vi "TwoCameraDisplayPanel.vi"() -> ()   [LabVIEW 2013]
uses:
  MvLVLib/MvCameraControl.lvlib
  MvLVLib/VIs/CreateGigEHandle.vi
  MvLVLib/VIs/CreateU3VHandle.vi
  <vilib>/picture/picture.llb/imagedata.ctl
panel:
  out "GenTLDeviceArray":T1(array[cluster])
  in  "image data 2":T2 caption="图像数据"
  in  "Rectangle 2":T3
  out "pFrameInfoEx out 2":T4
  in  "pConvertInfo In 2":T5
  out "nWidth 2":u32
  out "nHeight 2":u32
  out "PayloadSize 2":u32
  out "PixelFormat 2":u32
  out "handle out 2":u64
  in  "handle 2":u64
  out "Picture 2":picture
  in  "Device List 2":u16(ring)
  out "U3VDeviceArray":T6(array[cluster])
  out "GigEDeviceArray":T7(array[cluster])
  in  "pConvertInfo In":T5
  out "PixelFormat":u32
  out "handle out":u64
  in  "handle":u64
  in  "Rectangle":T3
  in  "image data":T2 caption="图像数据"
  out "Picture":picture
  out "PayloadSize":u32
  out "pFrameInfoEx out":T4
  out "nHeight":u32
  out "nWidth":u32
  out "Acquisision Flag":bool
  in  "Trigger Mode":bool
  in  "Continuous":bool
  out "打开标志":bool
  in  "stop":bool
  in  "Trigger Once":bool
  in  "Stop":bool
  in  "Start":bool
  in  "Open Device":bool
  in  "Close Device":bool
  in  "Refresh Devices":bool
  in  "Device List":u16(ring)
  # "Initialize"
  # "Acquisition"
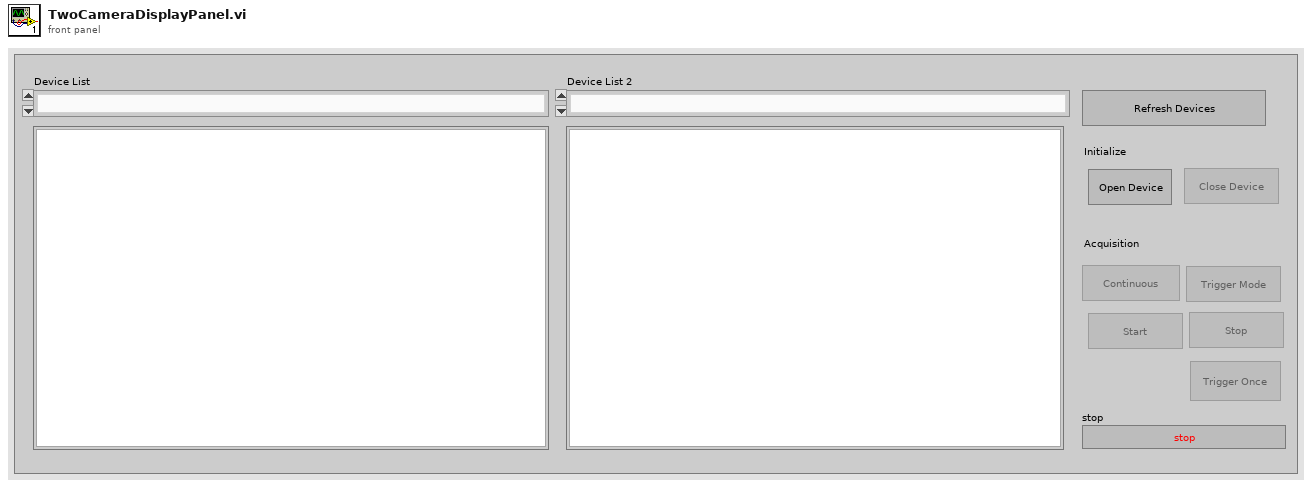
[diagram p1: front panel]
types:
  T1 = cluster{"nMajorVer":u16, "nMinorVer":u16, "nMacAddrHigh":u32, "nMacAddrLow":u32, "nTLayerType":u32, "nReserved0":u32, "nReserved1":u32, "nReserved2":u32, "nReserved3":u32, "chInterfaceID":string, "chVendorName":string, "chModelName":string, "chManufacturerInfo":string, "chDeviceVersion":string, "chSerialNumber":string, "chUserDefinedName":string, "chDeviceID":string, "nRes0":u32, "nRes1":u32, "nRes2":u32, "nRes3":u32, "nRes4":u32, "nRes5":u32, "nRes6":u32}[]
  T2 = typedef "imagedata.ctl" = cluster{"image type":i32, "image depth":i32, "image":u8[], "mask":u8[], "colors":u32[], "Rectangle":cluster{"left":i16, "top":i16, "right":i16, "bottom":i16}}
  T3 = cluster{"left":i16, "top":i16, "right":i16, "bottom":i16}
  T4 = cluster{"nWidth":u16, "nHeight":u16, "enPixelType":i32, "nFrameNum":u32, "nDevTimeStampHigh":u32, "nDevTimeStampLow":u32, "nReserved0":u32, "nHostTimeStamp":i64, "nFrameLen":u32, "nSecondCount]":u32, "nCycleCount":u32, "nCycleOffset":u32, "fGain":u32, "fExposureTime":u32, "nAverageBrightness":u32, "nRed":u32, "nGreen":u32, "nBlue":u32, "nFrameCounter":u32, "nTriggerIndex":u32, "nInput":u32, "nOutput":u32, "nOffsetX":u32, "nOffsetY":u32, "nReserved[0]":u32, "nReserved[1]":u32, "nReserved[2]":u32, "nReserved[3]":u32, "nReserved[4]":u32, "nReserved[5]":u32, "nReserved[6]":u32, "nReserved[7]":u32, "nReserved[8]":u32, "nReserved[9]":u32, "nReserved[10]":u32, "nReserved[11]":u32, "nReserved[12]":u32, "nReserved[13]":u32, "nReserved[14] 10":u32, "nReserved[15] 11":u32, "nReserved[16] 12":u32, "nReserved[17] 13":u32, "nReserved[18] 14":u32, "nReserved[19] 15":u32, "nReserved[20] 16":u32, "nReserved[21] 17":u32, "nReserved[22] 18":u32, "nReserved[23] 19":u32, "nReserved[24] 20":u32, "nReserved[25] 21":u32, "nReserved[26] 22":u32, "nReserved[27] 23":u32, "nReserved[28] 24":u32, "nReserved[29] 25":u32, "nReserved[30] 26":u32, "nReserved[31] 27":u32, "nReserved[32] 28":u32, "nReserved[33] 29":u32, "nReserved[34] 30":u32, "nReserved[35] 31":u32, "nReserved[36] 32":u32, "nReserved[37] 33":u32, "nReserved[38] 34":u32, "nReserved[39] 35":u32, "nReserved[40] 36":u32}
  T5 = cluster{"nWidth":u16, "nHeight":u16, "enSrcPixelType":u32, "nSrcDataLen":u32, "enDstPixelType":u32, "nDstLen":u32, "nDstBufferSize":u32, "nRes0":u32, "nRes1":u32, "nRes2":u32, "nRes3":u32}
  T6 = cluster{"nMajorVer":u16, "nMinorVer":u16, "nMacAddrHigh":u32, "nMacAddrLow":u32, "nTLayerType":u32, "nReserved0":u32, "nReserved1":u32, "nReserved2":u32, "nReserved3":u32, "CrtlInEndPoint":u8, "CrtlOutEndPoint":u8, "StreamEndPoint":u8, "EventEndPoint":u8, "idVendor":u16, "idProduct":u16, "nDeviceNumber":u32, "chDeviceGUID":string, "chVendorName":string, "chModelName":string, "chFamilyName":string, "chDeviceVersion":string, "chManufacturerName":string, "chSerialNumber":string, "chUserDefinedName":string, "nbcdUSB":u32, "nDeviceAddress":u32, "nRes0":u32, "nRes1":u32, "nResAlign":u32}[]
  T7 = cluster{"nMajorVer":u16, "nMinorVer":u16, "nMacAddrHigh":u32, "nMacAddrLow":u32, "nTLayerType":u32, "nReserved0":u32, "nReserved1":u32, "nReserved2":u32, "nReserved3":u32, "nIpCfgOption":u32, "nIpCfgCurrent":u32, "nCurrentIp":u32, "nCurrentSubNetMask":u32, "nDefaultGateWay":u32, "chManualfacturerName":string, "chModelName":string, "chDeviceVersion":string, "chManufacturerSpecificInfo":string, "chSerialNumber":string, "chUserDefinedName":string, "nNetExport":u32, "nRes0":u32, "nRes1":u32, "nRes2":u32, "nRes3":u32}[]
  T8 = enum8{"Enabled", "Disabled", "Disabled and Grayed Out"}
  T9 = cluster{"nMajorVer":u16, "nMinorVer":u16, "nMacAddrHigh":u32, "nMacAddrLow":u32, "nTLayerType":u32, "nReserved0":u32, "nReserved1":u32, "nReserved2":u32, "nReserved3":u32, "nIpCfgOption":u32, "nIpCfgCurrent":u32, "nCurrentIp":u32, "nCurrentSubNetMask":u32, "nDefaultGateWay":u32, "chManualfacturerName":string, "chModelName":string, "chDeviceVersion":string, "chManufacturerSpecificInfo":string, "chSerialNumber":string, "chUserDefinedName":string, "nNetExport":u32, "nRes0":u32, "nRes1":u32, "nRes2":u32, "nRes3":u32}
  T10 = cluster{"nMajorVer":u16, "nMinorVer":u16, "nMacAddrHigh":u32, "nMacAddrLow":u32, "nTLayerType":u32, "nReserved0":u32, "nReserved1":u32, "nReserved2":u32, "nReserved3":u32, "CrtlInEndPoint":u8, "CrtlOutEndPoint":u8, "StreamEndPoint":u8, "EventEndPoint":u8, "idVendor":u16, "idProduct":u16, "nDeviceNumber":u32, "chDeviceGUID":string, "chVendorName":string, "chModelName":string, "chFamilyName":string, "chDeviceVersion":string, "chManufacturerName":string, "chSerialNumber":string, "chUserDefinedName":string, "nbcdUSB":u32, "nDeviceAddress":u32, "nRes0":u32, "nRes1":u32, "nResAlign":u32}
  T11 = cluster{"nMajorVer":u16, "nMinorVer":u16, "nMacAddrHigh":u32, "nMacAddrLow":u32, "nTLayerType":u32, "nReserved0":u32, "nReserved1":u32, "nReserved2":u32, "nReserved3":u32, "chInterfaceID":string, "chVendorName":string, "chModelName":string, "chManufacturerInfo":string, "chDeviceVersion":string, "chSerialNumber":string, "chUserDefinedName":string, "chDeviceID":string, "nRes0":u32, "nRes1":u32, "nRes2":u32, "nRes3":u32, "nRes4":u32, "nRes5":u32, "nRes6":u32}
  T12 = cluster{"nCurValue":u32, "nMax":u32, "nMin":u32, "nInc":u32, "nReserved[0]":u32, "nReserved[1]":u32, "nReserved[2]":u32, "nReserved[3]":u32}
  T13 = cluster{"nCurValue":u32, "nSupportedNum":u32, "nSupportValue":u32[], "nReserved[0]":u32, "nReserved[1]":u32, "nReserved[2]":u32, "nReserved[3]":u32}
  T14 = cluster{"nWidth":u32, "nHeight":u32, "enSrcPixelType":u32, "nSrcDataLen":u32, "enDstPixelType":u32, "nDstLen":u32, "nDstBufferSize":u32, "nRes0":u32, "nRes1":u32, "nRes2":u32, "nRes3":u32}
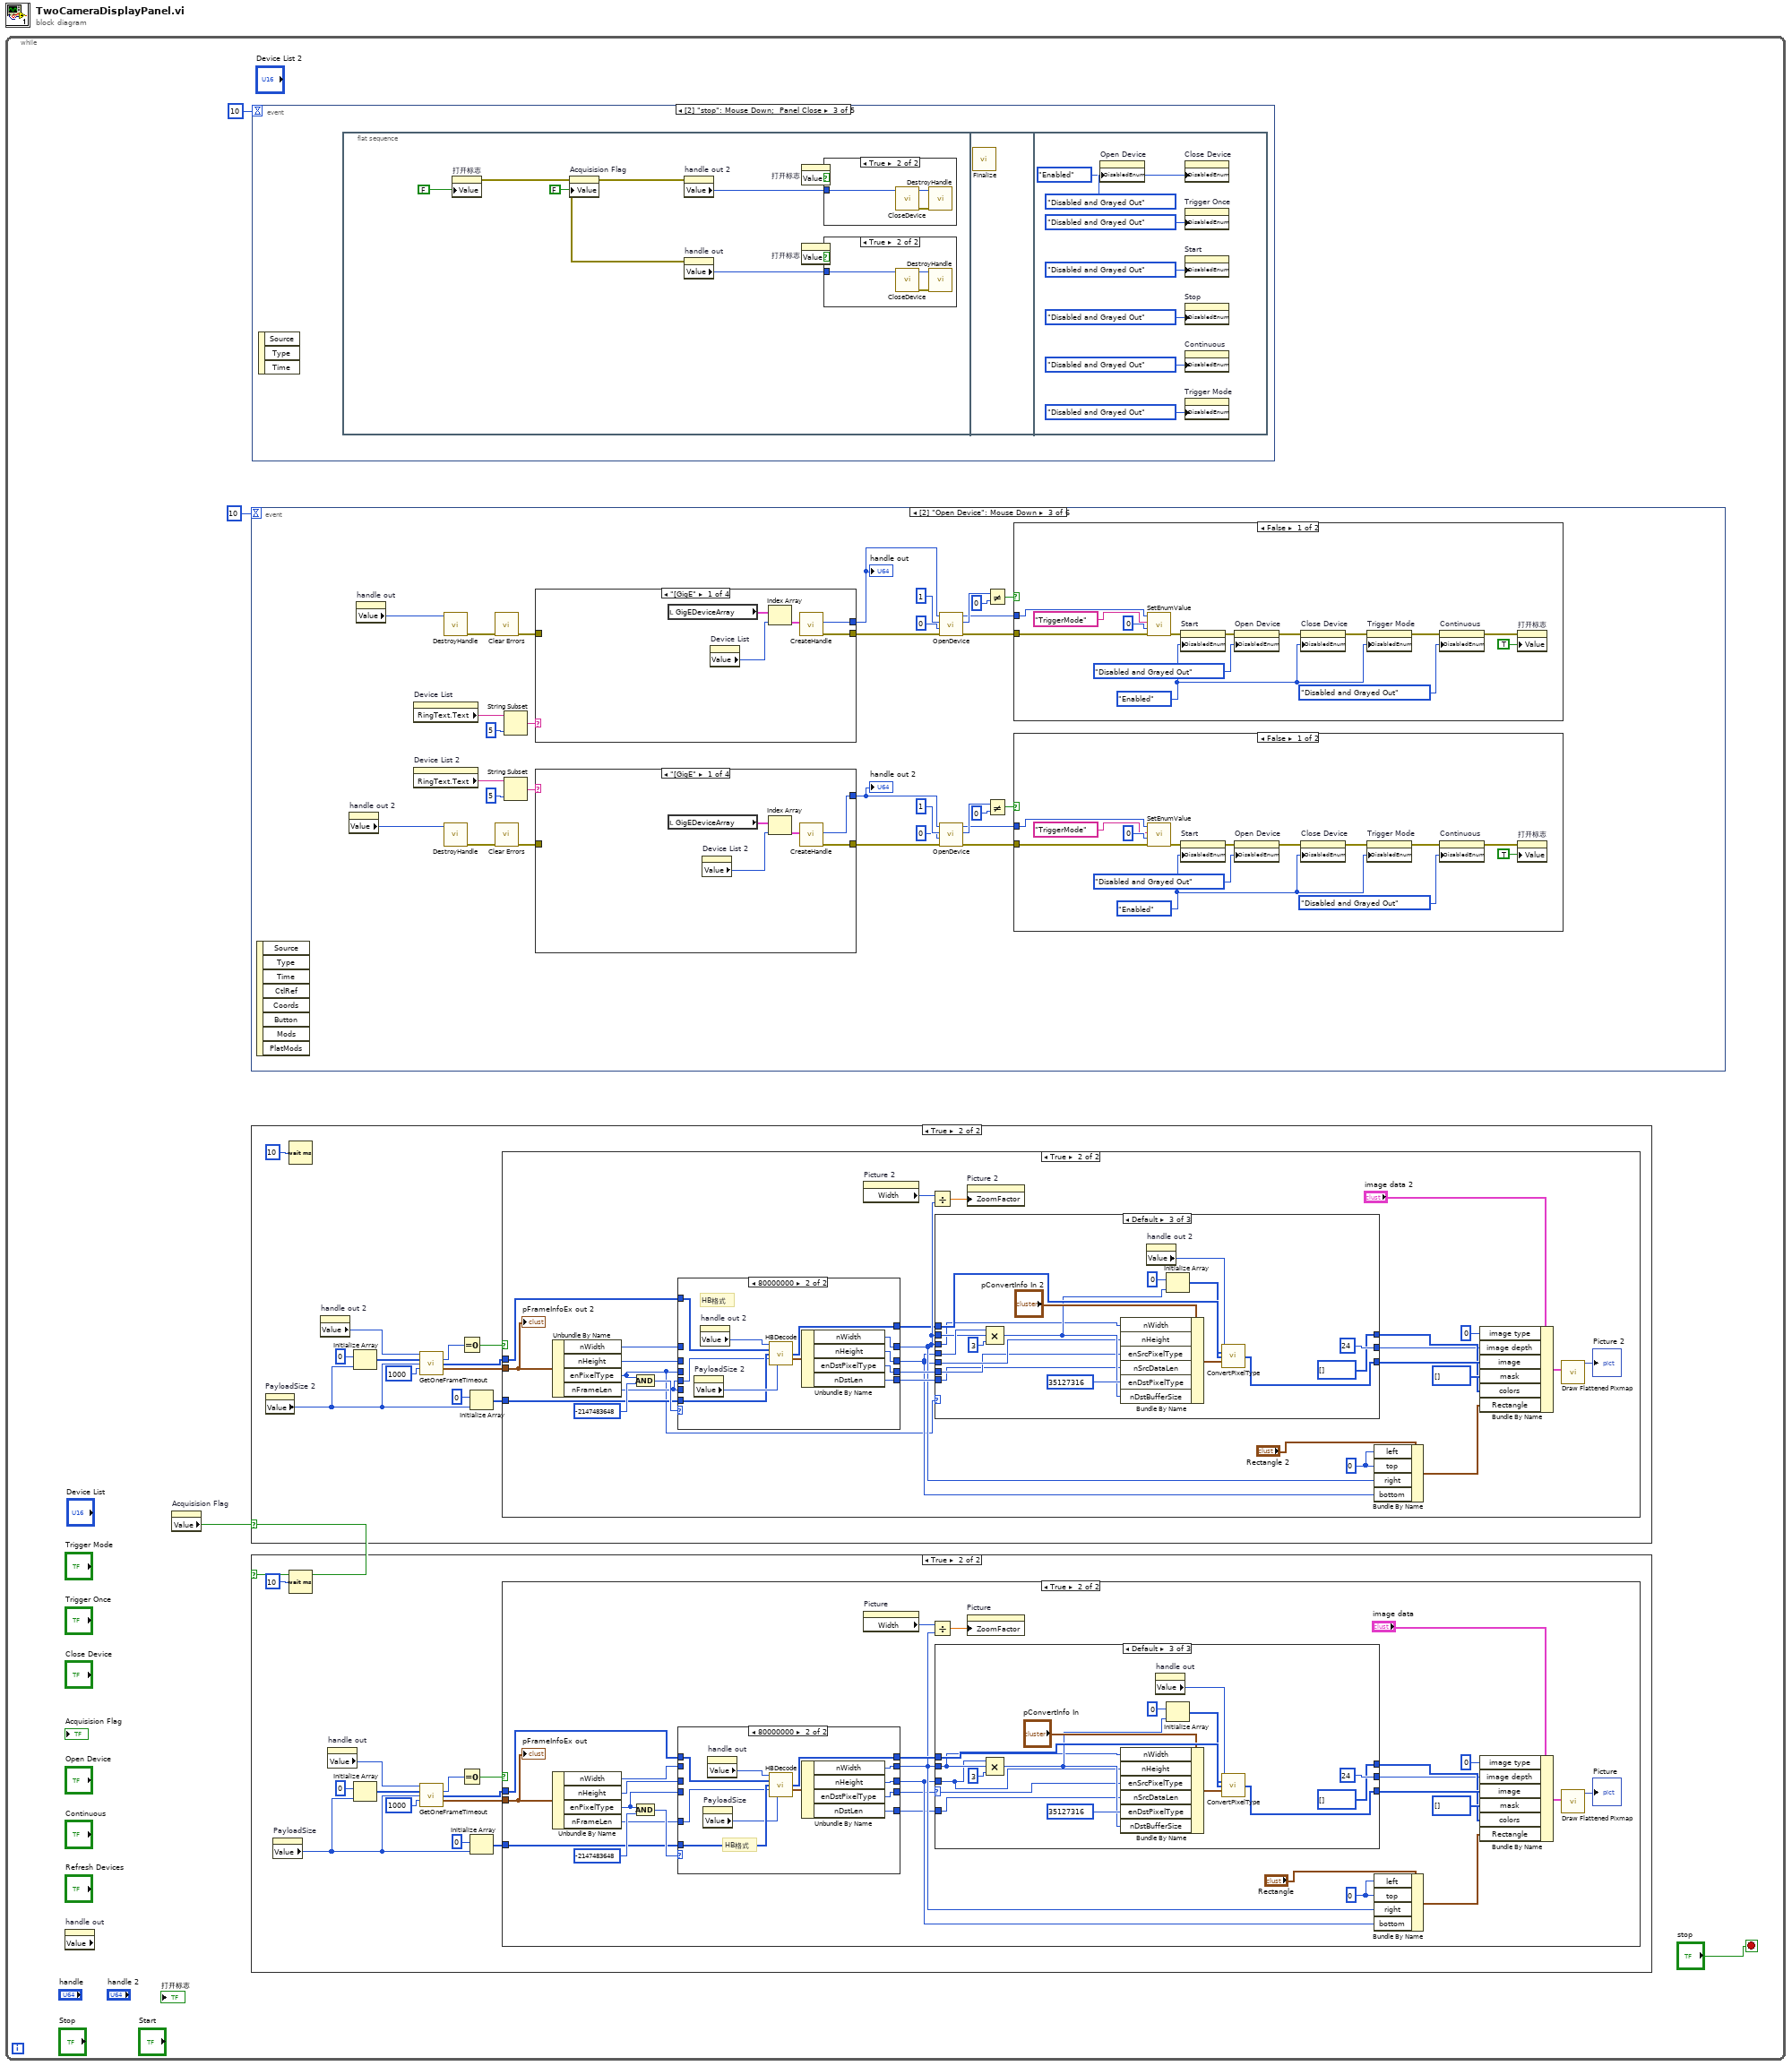
[diagram p0: block diagram]
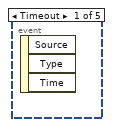
[diagram p2: hidden frame]
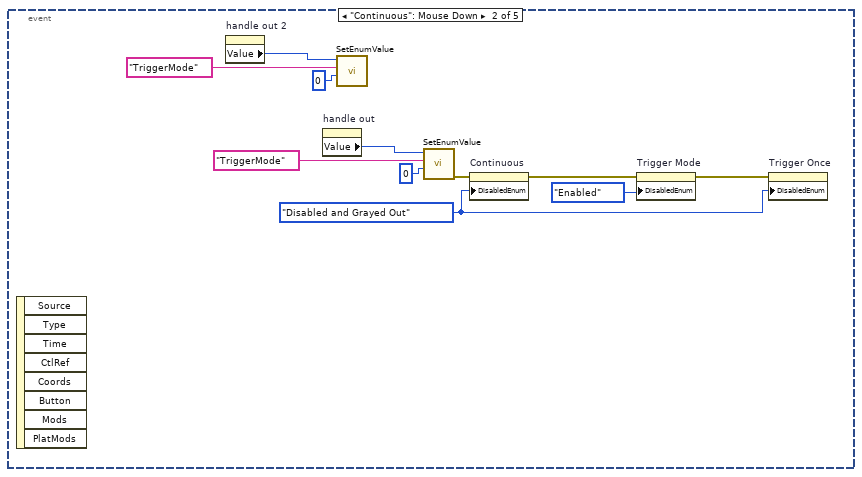
[diagram p3: hidden frame]
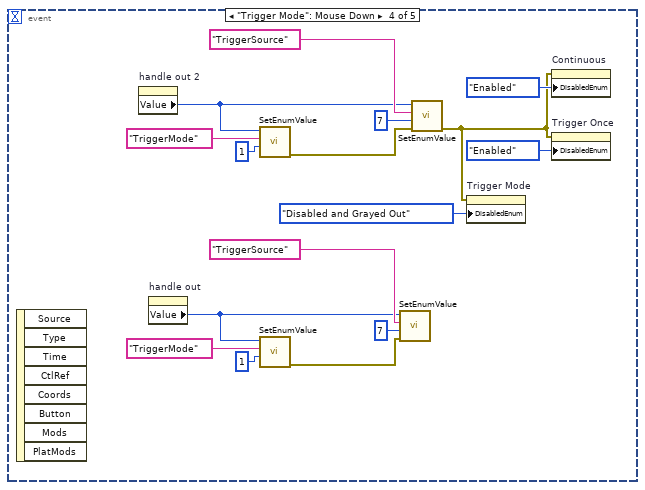
[diagram p6: hidden frame]
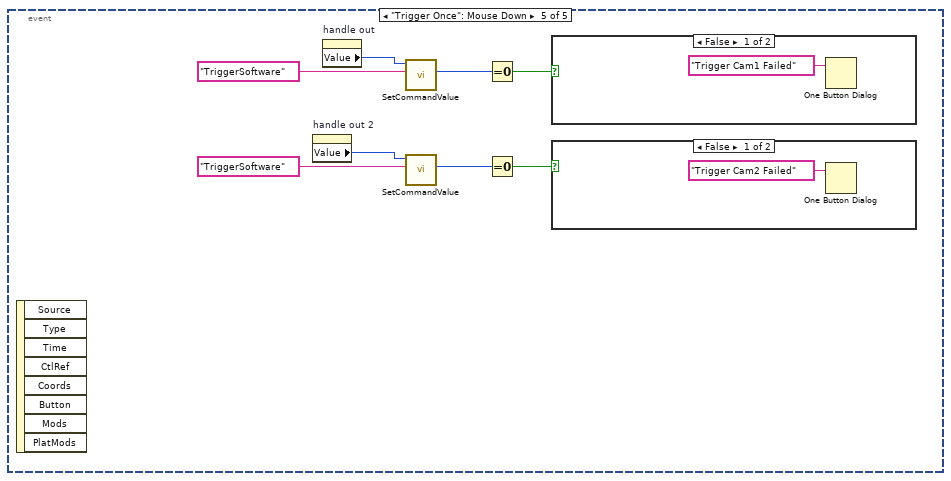
[diagram p7: hidden frame]
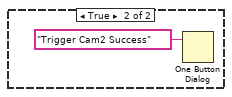
[diagram p8: hidden frame]
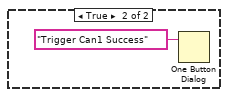
[diagram p9: hidden frame]
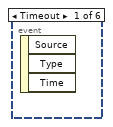
[diagram p10: hidden frame]
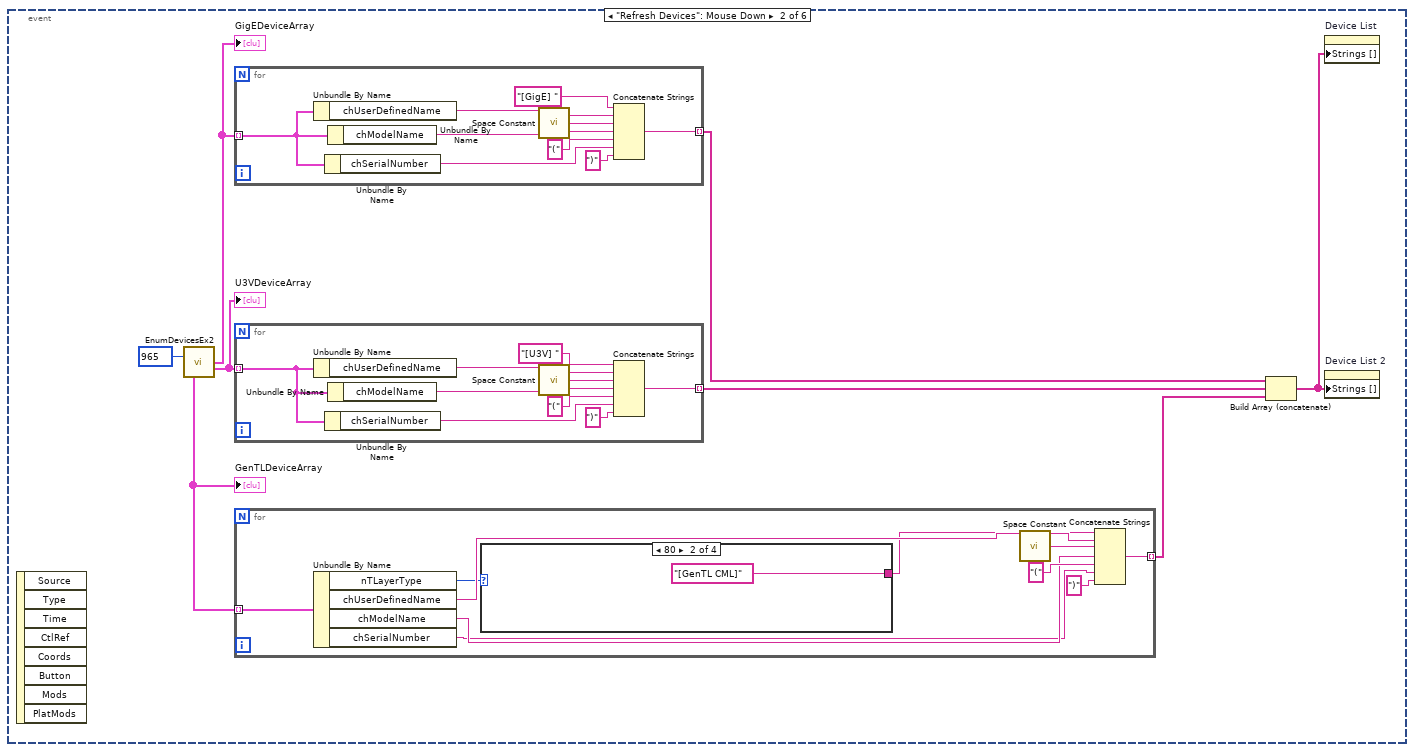
[diagram p11: hidden frame]
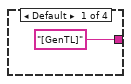
[diagram p12: hidden frame]
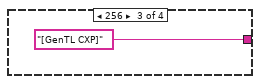
[diagram p13: hidden frame]
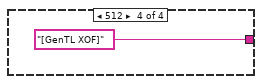
[diagram p14: hidden frame]
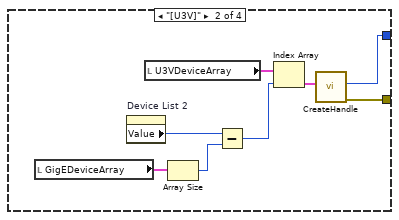
[diagram p15: hidden frame]
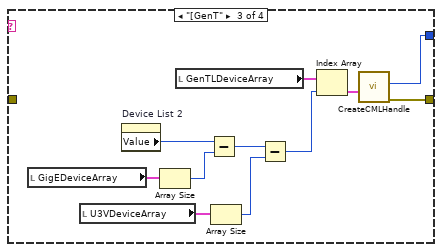
[diagram p16: hidden frame]
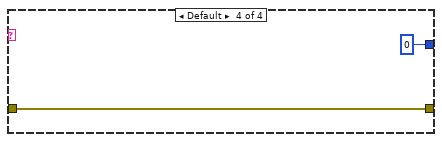
[diagram p17: hidden frame]
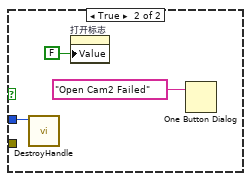
[diagram p18: hidden frame]
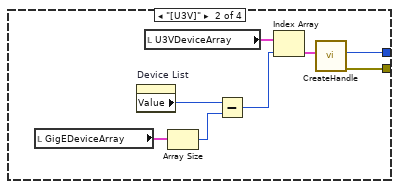
[diagram p19: hidden frame]
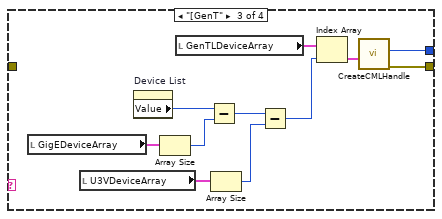
[diagram p20: hidden frame]
diagram:
  n1 = while {
    stop <- "stop" stop-if-true
    n2 = property on="handle out" class="DigNum (strict)" props=["Value"]() -> ()  [unwired: 2 in, 3 out]
    n3 = property on="Acquisision Flag" class="Bool (strict)"() -> ("Value"=w1:bool)  [unwired: 2 in, 2 out]
    n4 = event shown="[2] \"Open Device\": Mouse Down" {
      selector: _ -> [_ _ _ _ _ _]
      dyn-events: _ -> [_ _ _ _ _ _]
      timeout: 10 -> [_ _ _ _ _ _]
      event Timeout {
        n5 = event-data() -> ()  [unwired: 1 in, 3 out]
      }
      event "Refresh Devices": Mouse Down {
        n6 = event-data() -> ()  [unwired: 1 in, 8 out]
        n7 = call "EnumDevicesEx2.vi"("nLayerType"=u32 965) -> ("GigEDeviceArray"=w70:T7, "U3VDeviceArray"=w68:T6, "GenTLDevice"=w67:T1)  [unwired: 9 in, 3 out]
        "GigEDeviceArray" <- w70
        "U3VDeviceArray" <- w68
        "GenTLDeviceArray" <- w67
        n8 = for {
          tunnel: w70 -> [w98] mode=indexing
          tunnel: [w97] -> w65 mode=indexing
          n9 = Unbundle By Name(w98) -> ("chUserDefinedName"=w101:string)
          n10 = Unbundle By Name(w98) -> ("chSerialNumber"=w99:string)
          n11 = Unbundle By Name(w98) -> ("chModelName"=w100:string)
          n12 = call <vilib>:"Space Constant.vi"() -> ("String"=w104:string)
          n13 = Concatenate Strings("[GigE] " ("字符串"), w101, w104, w100, "(" ("字符串"), w99, ")" ("字符串")) -> (w97:string)
        }
        n14 = for {
          tunnel: w68 -> [w91] mode=indexing
          tunnel: [w88] -> w71 mode=indexing
          n15 = Unbundle By Name(w91) -> ("chUserDefinedName"=w95:string)
          n16 = Unbundle By Name(w91) -> ("chSerialNumber"=w90:string)
          n17 = Unbundle By Name(w91) -> ("chModelName"=w93:string)
          n18 = call <vilib>:"Space Constant.vi"() -> ("String"=w94:string)
          n19 = Concatenate Strings("[U3V] " ("字符串"), w95, w94, w93, "(" ("字符串"), w90, ")" ("字符串")) -> (w88:string)
        }
        n20 = for {
          tunnel: w67 -> [w79] mode=indexing
          tunnel: [w77] -> w66 mode=indexing
          n21 = Unbundle By Name(w79) -> ("nTLayerType"=w74:u32, "chUserDefinedName"=w82:string, "chModelName"=w76:string, "chSerialNumber"=w75:string)
          n22 = case shown="80" w74 {
            tunnel: ["[GenTL]" ("字符串") "[GenTL CML]" ("字符串") "[GenTL CXP]" ("字符串") "[GenTL XOF]" ("字符串")] -> w73
            frame Default {
            }
            frame 128 {
            }
            frame 256 {
            }
            frame 512 {
            }
          }
          n23 = call <vilib>:"Space Constant.vi"() -> ("String"=w81:string)
          n24 = Concatenate Strings(w73, w82, w81, w76, "(" ("字符串"), w75, ")" ("字符串")) -> (w77:string)
        }
        n25 = Build Array (concatenate)(w65, w71, w66) -> (w69:string[])
        n26 = property on="Device List" class="Ring (strict)"("Strings []"=w69) -> ()  [unwired: 2 in, 2 out]
        n27 = property on="Device List 2" class="Ring (strict)"("Strings []"=w69) -> ()  [unwired: 2 in, 2 out]
      }
      event "Open Device": Mouse Down {
        n28 = event-data() -> ()  [unwired: 1 in, 8 out]
        n29 = property on="handle out 2" class="DigNum (strict)"() -> ("Value"=w111:u64)  [unwired: 2 in, 2 out]
        n30 = property on="handle out" class="DigNum (strict)"() -> ("Value"=w127:u64)  [unwired: 2 in, 2 out]
        n31 = property on="Device List" class="Ring (strict)"() -> ("RingText.Text"=w124:string)  [unwired: 2 in, 2 out]
        n32 = property on="Device List 2" class="Ring (strict)"() -> ("RingText.Text"=w109:string)  [unwired: 2 in, 2 out]
        n33 = call "DestroyHandle.vi"("handle"=w127) -> ("error out"=w126:errorcluster)  [unwired: 9 in, 1 out]
        n34 = call "DestroyHandle.vi"("handle"=w111) -> ("error out"=w112:errorcluster)  [unwired: 9 in, 1 out]
        n35 = call <vilib>:"Clear Errors.vi"("error in (no error)"=w126) -> ("error out"=w120:errorcluster)  [unwired: 5 in, 1 out]
        n36 = call <vilib>:"Clear Errors.vi"("error in (no error)"=w112) -> ("error out"=w105:errorcluster)  [unwired: 5 in, 1 out]
        n37 = String Subset(string=w124, length (rest)=5 ("长度（剩余）")) -> (substring=w123:string)  [unwired: 1 in]
        n38 = String Subset(string=w109, length (rest)=5 ("长度（剩余）")) -> (substring=w108:string)  [unwired: 1 in]
        n39 = case shown="\"[GigE\"" w123 {
          tunnel: [w181 w187 w199 w203] -> w122
          tunnel: [w180 w186 w198 u64 0 ("handle")] -> w121
          tunnel: w120 -> [_ _ _ w203]
          frame "[GigE" {
            n40 = local read "GigEDeviceArray"() -> (w179:T7)
            n41 = property on="Device List" class="Ring (strict)"() -> ("Value"=w182:u16)  [unwired: 2 in, 2 out]
            n42 = Index Array(array=w179, index=w182) -> (element=w178:T9)
            n43 = call-poly "CreateHandle.vi"("GigEDevice"=w178) -> ("error out"=w181:errorcluster, "handle"=w180:u64)  [unwired: 7 in, 1 out]
          }
          frame "[U3V]" {
            n44 = local read "GigEDeviceArray"() -> (w184:T7)
            n45 = property on="Device List" class="Ring (strict)"() -> ("Value"=w190:u16)  [unwired: 2 in, 2 out]
            n46 = local read "U3VDeviceArray"() -> (w185:T6)
            n47 = Array Size(array=w184) -> (size(s)=w189:i32)
            n48 = Subtract(x=w190, y=w189) -> (x-y=w188:i32)
            n49 = Index Array(array=w185, index=w188) -> (element=w183:T10)
            n50 = call-poly "CreateHandle.vi"("U3VDevice"=w183) -> ("error out"=w187:errorcluster, "handle"=w186:u64)  [unwired: 7 in, 1 out]
          }
          frame "[GenT" {
            n51 = local read "GigEDeviceArray"() -> (w192:T7)
            n52 = local read "U3VDeviceArray"() -> (w191:T6)
            n53 = property on="Device List" class="Ring (strict)"() -> ("Value"=w201:u16)  [unwired: 2 in, 2 out]
            n54 = Array Size(array=w192) -> (size(s)=w200:i32)
            n55 = local read "GenTLDeviceArray"() -> (w197:T1)
            n56 = Subtract(x=w201, y=w200) -> (x-y=w196:i32)
            n57 = Array Size(array=w191) -> (size(s)=w195:i32)
            n58 = Subtract(x=w196, y=w195) -> (x-y=w194:i32)
            n59 = Index Array(array=w197, index=w194) -> (element=w193:T11)
            n60 = call "CreateCMLHandle.vi"("GenTLCMLDevice"=w193) -> ("error out"=w199:errorcluster, "handle"=w198:u64)  [unwired: 7 in, 1 out]
          }
          frame Default {
          }
        }
        "handle out" <- w121
        n61 = case shown="\"[GigE\"" w108 {
          tunnel: [w138 w144 w156 w160] -> w106
          tunnel: [w137 w143 w155 u64 0 ("handle")] -> w107
          tunnel: w105 -> [_ _ _ w160]
          frame "[GigE" {
            n62 = local read "GigEDeviceArray"() -> (w136:T7)
            n63 = property on="Device List 2" class="Ring (strict)"() -> ("Value"=w139:u16)  [unwired: 2 in, 2 out]
            n64 = Index Array(array=w136, index=w139) -> (element=w135:T9)
            n65 = call-poly "CreateHandle.vi"("GigEDevice"=w135) -> ("error out"=w138:errorcluster, "handle"=w137:u64)  [unwired: 7 in, 1 out]
          }
          frame "[U3V]" {
            n66 = local read "GigEDeviceArray"() -> (w141:T7)
            n67 = property on="Device List 2" class="Ring (strict)"() -> ("Value"=w147:u16)  [unwired: 2 in, 2 out]
            n68 = local read "U3VDeviceArray"() -> (w142:T6)
            n69 = Array Size(array=w141) -> (size(s)=w146:i32)
            n70 = Subtract(x=w147, y=w146) -> (x-y=w145:i32)
            n71 = Index Array(array=w142, index=w145) -> (element=w140:T10)
            n72 = call-poly "CreateHandle.vi"("U3VDevice"=w140) -> ("error out"=w144:errorcluster, "handle"=w143:u64)  [unwired: 7 in, 1 out]
          }
          frame "[GenT" {
            n73 = local read "GigEDeviceArray"() -> (w149:T7)
            n74 = local read "U3VDeviceArray"() -> (w148:T6)
            n75 = property on="Device List 2" class="Ring (strict)"() -> ("Value"=w158:u16)  [unwired: 2 in, 2 out]
            n76 = Array Size(array=w149) -> (size(s)=w157:i32)
            n77 = local read "GenTLDeviceArray"() -> (w154:T1)
            n78 = Subtract(x=w158, y=w157) -> (x-y=w153:i32)
            n79 = Array Size(array=w148) -> (size(s)=w152:i32)
            n80 = Subtract(x=w153, y=w152) -> (x-y=w151:i32)
            n81 = Index Array(array=w154, index=w151) -> (element=w150:T11)
            n82 = call "CreateCMLHandle.vi"("GenTLCMLDevice"=w150) -> ("error out"=w156:errorcluster, "handle"=w155:u64)  [unwired: 7 in, 1 out]
          }
          frame Default {
          }
        }
        "handle out 2" <- w107
        n83 = call "OpenDevice.vi"("error in (no error)"=w122, "nSwitchoverKey"=u16 0, "nAccessMode"=u32 1, "handle"=w121) -> ("error out"=w130:errorcluster, "return"=w129:i32, "handle out"=w128:u64)  [unwired: 5 in]
        n84 = call "OpenDevice.vi"("error in (no error)"=w106, "nSwitchoverKey"=u16 0, "nAccessMode"=u32 1, "handle"=w107) -> ("error out"=w115:errorcluster, "return"=w114:i32, "handle out"=w113:u64)  [unwired: 5 in]
        n85 = Not Equal?(x=w129, y=0) -> (x != y?=w133:bool)
        n86 = Not Equal?(x=w114, y=0) -> (x != y?=w118:bool)
        n87 = case shown="False" w133 {
          tunnel: w128 -> [w205 w218]
          tunnel: w130 -> [w206 _]
          frame False {
            w204 = T8."Enabled" ("禁用")
            n88 = call "SetEnumValue.vi"("error in (no error)"=w206, "nValue"=u32 0, "strKey"="TriggerMode", "handle"=w205) -> ("error out"=w216:errorcluster)  [unwired: 5 in, 2 out]
            n89 = property on="Start" class="Bool"(error in=w216, "DisabledEnum"=w204) -> (error out=w214:errorcluster)  [unwired: 1 in, 1 out]
            n90 = property on="Open Device" class="Bool"(error in=w214, "DisabledEnum"=T8."Disabled and Grayed Out" ("禁用")) -> (error out=w213:errorcluster)  [unwired: 1 in, 1 out]
            n91 = property on="Close Device" class="Bool"(error in=w213, "DisabledEnum"=w204) -> (error out=w211:errorcluster)  [unwired: 1 in, 1 out]
            n92 = property on="Trigger Mode" class="Bool"(error in=w211, "DisabledEnum"=w204) -> (error out=w209:errorcluster)  [unwired: 1 in, 1 out]
            n93 = property on="Continuous" class="Bool"(error in=w209, "DisabledEnum"=T8."Disabled and Grayed Out" ("禁用")) -> (error out=w207:errorcluster)  [unwired: 1 in, 1 out]
            n94 = property on="打开标志" class="Bool (strict)"(error in=w207, "Value"=TRUE ("布尔")) -> ()  [unwired: 1 in, 2 out]
          }
          frame True {
            n95 = call "DestroyHandle.vi"("handle"=w218) -> ()  [unwired: 9 in, 2 out]
            n96 = property on="打开标志" class="Bool (strict)"("Value"=FALSE) -> ()  [unwired: 2 in, 2 out]
            n97 = One Button Dialog(message="Open Cam1 Failed") -> ()  [unwired: 1 in, 1 out]
          }
        }
        n98 = case shown="False" w118 {
          tunnel: w113 -> [w162 w175]
          tunnel: w115 -> [w163 _]
          frame False {
            w161 = T8."Enabled" ("禁用")
            n99 = call "SetEnumValue.vi"("error in (no error)"=w163, "nValue"=u32 0, "strKey"="TriggerMode", "handle"=w162) -> ("error out"=w173:errorcluster)  [unwired: 5 in, 2 out]
            n100 = property on="Start" class="Bool"(error in=w173, "DisabledEnum"=w161) -> (error out=w171:errorcluster)  [unwired: 1 in, 1 out]
            n101 = property on="Open Device" class="Bool"(error in=w171, "DisabledEnum"=T8."Disabled and Grayed Out" ("禁用")) -> (error out=w170:errorcluster)  [unwired: 1 in, 1 out]
            n102 = property on="Close Device" class="Bool"(error in=w170, "DisabledEnum"=w161) -> (error out=w168:errorcluster)  [unwired: 1 in, 1 out]
            n103 = property on="Trigger Mode" class="Bool"(error in=w168, "DisabledEnum"=w161) -> (error out=w166:errorcluster)  [unwired: 1 in, 1 out]
            n104 = property on="Continuous" class="Bool"(error in=w166, "DisabledEnum"=T8."Disabled and Grayed Out" ("禁用")) -> (error out=w164:errorcluster)  [unwired: 1 in, 1 out]
            n105 = property on="打开标志" class="Bool (strict)"(error in=w164, "Value"=TRUE ("布尔")) -> ()  [unwired: 1 in, 2 out]
          }
          frame True {
            n106 = call "DestroyHandle.vi"("handle"=w175) -> ()  [unwired: 9 in, 2 out]
            n107 = property on="打开标志" class="Bool (strict)"("Value"=FALSE) -> ()  [unwired: 2 in, 2 out]
            n108 = One Button Dialog(message="Open Cam2 Failed") -> ()  [unwired: 1 in, 1 out]
          }
        }
      }
      event "Close Device": Mouse Down {
        w222 = T8."Disabled and Grayed Out" ("禁用")
        n109 = event-data() -> ()  [unwired: 1 in, 8 out]
        n110 = property on="打开标志" class="Bool (strict)"("Value"=FALSE ("打开标志")) -> (error out=w227:errorcluster)  [unwired: 2 in, 1 out]
        n111 = property on="Acquisision Flag" class="Bool (strict)"(error in=w227, "Value"=FALSE ("采集标志")) -> (error out=w221:errorcluster)  [unwired: 1 in, 1 out]
        n112 = property on="Open Device" class="Bool"("DisabledEnum"=T8."Enabled" ("禁用")) -> (error out=w229:errorcluster)  [unwired: 2 in, 1 out]
        n113 = property on="Close Device" class="Bool"(error in=w229, "DisabledEnum"=w222) -> ()  [unwired: 1 in, 2 out]
        n114 = property on="Start" class="Bool"("DisabledEnum"=w222) -> ()  [unwired: 2 in, 2 out]
        n115 = property on="Stop" class="Bool"("DisabledEnum"=w222) -> ()  [unwired: 2 in, 2 out]
        n116 = property on="Trigger Once" class="Bool"("DisabledEnum"=w222) -> ()  [unwired: 2 in, 2 out]
        n117 = property on="Continuous" class="Bool"("DisabledEnum"=w222) -> ()  [unwired: 2 in, 2 out]
        n118 = property on="Trigger Mode" class="Bool"("DisabledEnum"=w222) -> ()  [unwired: 2 in, 2 out]
        n119 = property on="handle out" class="DigNum (strict)"(error in=w221) -> ("Value"=w223:u64)  [unwired: 1 in, 2 out]
        n120 = property on="handle out 2" class="DigNum (strict)"(error in=w221) -> ("Value"=w231:u64)  [unwired: 1 in, 2 out]
        n121 = call "CloseDevice.vi"("handle"=w223) -> ("error out"=w225:errorcluster, "handle out"=w224:u64)  [unwired: 8 in, 1 out]
        n122 = call "CloseDevice.vi"("handle"=w231) -> ("error out"=w233:errorcluster, "handle out"=w232:u64)  [unwired: 8 in, 1 out]
        n123 = call "DestroyHandle.vi"("error in (no error)"=w225, "handle"=w224) -> ()  [unwired: 8 in, 2 out]
        n124 = call "DestroyHandle.vi"("error in (no error)"=w233, "handle"=w232) -> ()  [unwired: 8 in, 2 out]
      }
      event "Start": Mouse Down {
        n125 = event-data() -> ()  [unwired: 1 in, 8 out]
        n126 = property on="handle out 2" class="DigNum (strict)"() -> ("Value"=w234:u64)  [unwired: 2 in, 2 out]
        n127 = property on="handle out" class="DigNum (strict)"() -> ("Value"=w249:u64)  [unwired: 2 in, 2 out]
        n128 = call "GetIntValue.vi"("strKey"="PayloadSize", "handle"=w234) -> ("error out"=w244:errorcluster, "pIntValue out"=w240:T12, "handle out"=w237:u64)  [unwired: 6 in, 1 out]
        n129 = call "GetIntValue.vi"("strKey"="PayloadSize", "handle"=w249) -> ("error out"=w259:errorcluster, "pIntValue out"=w255:T12, "handle out"=w252:u64)  [unwired: 6 in, 1 out]
        n130 = Unbundle By Name(w240) -> ("nCurValue"=→"PayloadSize 2":u32)
        n131 = Unbundle By Name(w255) -> ("nCurValue"=→"PayloadSize":u32)
        n132 = call "GetEnumValue.vi"("error in (no error)"=w244, "strKey"="PixelFormat", "handle"=w237) -> ("error out"=w243:errorcluster, "pEnumValue out"=w245:T13, "handle out"=w236:u64)  [unwired: 5 in, 1 out]
        n133 = call "GetEnumValue.vi"("error in (no error)"=w259, "strKey"="PixelFormat", "handle"=w252) -> ("error out"=w258:errorcluster, "pEnumValue out"=w260:T13, "handle out"=w251:u64)  [unwired: 5 in, 1 out]
        n134 = Unbundle By Name(w245) -> ("nCurValue"=→"PixelFormat 2":u32)
        n135 = Unbundle By Name(w260) -> ("nCurValue"=→"PixelFormat":u32)
        n136 = call "StartGrabbing.vi"("error in (no error)"=w243, "handle"=w236) -> ("error out"=w242:errorcluster, "function return"=w248:i32, "handle out"=w235:u64)  [unwired: 7 in]
        n137 = call "StartGrabbing.vi"("error in (no error)"=w258, "handle"=w251) -> ("error out"=w257:errorcluster, "function return"=w263:i32, "handle out"=w250:u64)  [unwired: 7 in]
        n138 = Not Equal To 0?(x=w248) -> (x != 0?=w247:bool)
        n139 = Not Equal To 0?(x=w263) -> (x != 0?=w262:bool)
        n140 = case shown="False" w247 {
          tunnel: w234 -> [_ _]
          tunnel: w242 -> [w268 _]
          tunnel: w235 -> [w267 _]
          frame False {
            n141 = call "GetIntValue.vi"("error in (no error)"=w268, "strKey"="Width", "handle"=w267) -> ("error out"=w274:errorcluster, "pIntValue out"=w269:T12, "handle out"=w266:u64)  [unwired: 5 in, 1 out]
            n142 = Unbundle By Name(w269) -> ("nCurValue"=→"nWidth 2":u32)
            n143 = property on="Stop" class="Bool"("DisabledEnum"=T8."Enabled" ("禁用")) -> (error out=w270:errorcluster)  [unwired: 2 in, 1 out]
            n144 = property on="Continuous" class="Bool"(error in=w270) -> (error out=w279:errorcluster, "DisabledEnum"=w280:T8)  [unwired: 1 in, 1 out]
            n145 = call "GetIntValue.vi"("error in (no error)"=w274, "strKey"="Height", "handle"=w266) -> ("error out"=w265:errorcluster, "pIntValue out"=w272:T12)  [unwired: 5 in, 2 out]
            n146 = Unbundle By Name(w272) -> ("nCurValue"=→"nHeight 2":u32)
            n147 = Equal To 0?(x=w280) -> (x = 0?=w281:bool)
            n148 = case shown="True" w281 {
              tunnel: w279 -> [w284 w287]
              tunnel: [w283 w286] -> w278
              frame False {
                n149 = property on="Trigger Once" class="Bool"(error in=w284, "DisabledEnum"=T8."Disabled and Grayed Out" ("禁用")) -> (error out=w283:errorcluster)  [unwired: 1 in, 1 out]
              }
              frame True {
                n150 = property on="Trigger Once" class="Bool"(error in=w287, "DisabledEnum"=T8."Enabled" ("禁用")) -> (error out=w286:errorcluster)  [unwired: 1 in, 1 out]
              }
            }
            n151 = property on="Start" class="Bool"(error in=w265, "DisabledEnum"=T8."Disabled and Grayed Out" ("禁用")) -> ()  [unwired: 1 in, 2 out]
            n152 = property on="Acquisision Flag" class="Bool (strict)"(error in=w278, "Value"=TRUE ("采集标志")) -> ()  [unwired: 1 in, 2 out]
          }
          frame True {
            n153 = One Button Dialog(message="Start Cam2 Failed") -> ()  [unwired: 1 in, 1 out]
          }
        }
        n154 = case shown="False" w262 {
          tunnel: w249 -> [_ _]
          tunnel: w257 -> [w292 _]
          tunnel: w250 -> [w291 _]
          frame False {
            n155 = call "GetIntValue.vi"("error in (no error)"=w292, "strKey"="Width", "handle"=w291) -> ("error out"=w299:errorcluster, "pIntValue out"=w293:T12, "handle out"=w290:u64)  [unwired: 5 in, 1 out]
            n156 = Unbundle By Name(w293) -> ("nCurValue"=→"nWidth":u32)
            n157 = call "GetIntValue.vi"("error in (no error)"=w299, "strKey"="Height", "handle"=w290) -> ("error out"=w298:errorcluster, "pIntValue out"=w296:T12)  [unwired: 5 in, 2 out]
            n158 = Unbundle By Name(w296) -> ("nCurValue"=→"nHeight":u32)
            n159 = property on="Start" class="Bool"(error in=w298, "DisabledEnum"=T8."Disabled and Grayed Out" ("禁用")) -> (error out=w308:errorcluster)  [unwired: 1 in, 1 out]
            n160 = property on="Stop" class="Bool"(error in=w308, "DisabledEnum"=T8."Enabled" ("禁用")) -> (error out=w294:errorcluster)  [unwired: 1 in, 1 out]
            n161 = property on="Continuous" class="Bool"(error in=w294) -> (error out=w304:errorcluster, "DisabledEnum"=w305:T8)  [unwired: 1 in, 1 out]
            n162 = Equal To 0?(x=w305) -> (x = 0?=w306:bool)
            n163 = case shown="True" w306 {
              tunnel: w304 -> [w311 w314]
              tunnel: [w310 w313] -> w303
              frame False {
                n164 = property on="Trigger Once" class="Bool"(error in=w311, "DisabledEnum"=T8."Disabled and Grayed Out" ("禁用")) -> (error out=w310:errorcluster)  [unwired: 1 in, 1 out]
              }
              frame True {
                n165 = property on="Trigger Once" class="Bool"(error in=w314, "DisabledEnum"=T8."Enabled" ("禁用")) -> (error out=w313:errorcluster)  [unwired: 1 in, 1 out]
              }
            }
            n166 = property on="Acquisision Flag" class="Bool (strict)"(error in=w303, "Value"=TRUE ("采集标志")) -> ()  [unwired: 1 in, 2 out]
          }
          frame True {
            n167 = One Button Dialog(message="Start Cam1 Failed") -> ()  [unwired: 1 in, 1 out]
          }
        }
      }
      event "Stop": Mouse Down {
        n168 = event-data() -> ()  [unwired: 1 in, 8 out]
        n169 = property on="Acquisision Flag" class="Bool (strict)"("Value"=FALSE ("采集标志")) -> (error out=w318:errorcluster)  [unwired: 2 in, 1 out]
        n170 = property on="handle out" class="DigNum (strict)"(error in=w318) -> ("Value"=w326:u64)  [unwired: 1 in, 2 out]
        n171 = property on="handle out 2" class="DigNum (strict)"(error in=w318) -> (error out=w317:errorcluster, "Value"=w319:u64)  [unwired: 1 in, 1 out]
        n172 = call "StopGrabbing.vi"("handle"=w326) -> ()  [unwired: 8 in, 3 out]
        n173 = call "StopGrabbing.vi"("handle"=w319) -> ()  [unwired: 8 in, 3 out]
        n174 = property on="Start" class="Bool"(error in=w317, "DisabledEnum"=T8."Enabled" ("禁用")) -> (error out=w321:errorcluster)  [unwired: 1 in, 1 out]
        n175 = property on="Stop" class="Bool"(error in=w321, "DisabledEnum"=T8."Disabled and Grayed Out" ("禁用")) -> (error out=w320:errorcluster)  [unwired: 1 in, 1 out]
        n176 = property on="Trigger Once" class="Bool"(error in=w320, "DisabledEnum"=T8."Disabled and Grayed Out" ("禁用")) -> ()  [unwired: 1 in, 2 out]
      }
    }
    n177 = case shown="True" w1 {
      frame False {
      }
      frame True {
        n178 = property on="PayloadSize 2" class="DigNum (strict)"() -> ("Value"=w327:u32)  [unwired: 2 in, 2 out]
        n179 = Wait (ms)(milliseconds to wait=u32 10 ("等待时间（毫秒）")) -> ()  [unwired: 1 out]
        n180 = property on="handle out 2" class="DigNum (strict)"() -> ("Value"=w332:u64)  [unwired: 2 in, 2 out]
        n181 = Initialize Array(u8 0 ("元素"), w327) -> (w330:u8[])
        n182 = call "GetOneFrameTimeout.vi"("handle"=w332, "pData"=w330, "nDataSize"=w327, "nMsec"=1000) -> ("function return"=w335:i32, "pData Out"=w334:u8[], "pFrameInfoEx out"=w333:T4)  [unwired: 7 in, 2 out]
        n183 = Equal To 0?(x=w335) -> (x = 0?=w337:bool)
        n184 = Initialize Array(u8 0 ("元素"), w327) -> (w328:u8[])
        n185 = case shown="True" w337 {
          tunnel: w334 -> [_ w348]
          tunnel: w333 -> [_ w352]
          tunnel: w328 -> [_ w349]
          frame False {
          }
          frame True {
            w365 = i16 0 ("left")
            n186 = Unbundle By Name(w352) -> ("nWidth"=w347:u16, "nHeight"=w346:u16, "enPixelType"=w339:i32, "nFrameLen"=w345:u32)
            n187 = Compound Arithmetic op=AND(w339, -2147483648 ("value")) -> (w350:i32)
            n188 = case shown="80000000" w350 {
              tunnel: [w370 w378] -> w340
              tunnel: [w369 w377] -> w342
              tunnel: [w368 w376] -> w341
              tunnel: [w366 w375] -> w344
              tunnel: [w367 w374] -> w343
              tunnel: w349 -> [_ w373]
              tunnel: w348 -> [w370 w372]
              tunnel: w345 -> [_ w371]
              tunnel: w347 -> [w369 _]
              tunnel: w346 -> [w368 _]
              tunnel: w345 -> [w367 _]
              tunnel: w339 -> [w366 _]
              frame Default {
              }
              frame -2147483648 {
                # "HB格式"
                n189 = property on="PayloadSize 2" class="DigNum (strict)"() -> ("Value"=w380:u32)  [unwired: 2 in, 2 out]
                n190 = property on="handle out 2" class="DigNum (strict)"() -> ("Value"=w381:u64)  [unwired: 2 in, 2 out]
                n191 = call "HBDecode.vi"("handle"=w381, "pSrcData"=w372, "pDstBuf In"=w373, "SrcDataLen"=w371, "DstBufferSize"=w380) -> ("pDstBuf Out"=w378:u8[], "pHBDecode Out"=w379:T14)  [unwired: 6 in, 3 out]
                n192 = Unbundle By Name(w379) -> ("nWidth"=w377:u32, "nHeight"=w376:u32, "enDstPixelType"=w375:u32, "nDstLen"=w374:u32)
              }
            }
            n193 = property on="Picture 2" class="Pict"() -> ("Width"=w360:u32)  [unwired: 2 in, 2 out]
            n194 = Divide(x=w360, y=w342) -> (x/y=w359:dbl)
            n195 = case shown="Default" w339 {
              tunnel: w340 -> [w384 w399 w414]
              tunnel: w341 -> [_ _ w411]
              tunnel: w342 -> [_ _ w410]
              tunnel: [w384 w399 w404] -> w358
              tunnel: [8 24 24] -> w353
              tunnel: [w382 i32[] [] i32[] []] -> w357
              tunnel: w342 -> [_ _ w403]
              tunnel: w341 -> [_ _ w402]
              tunnel: w344 -> [_ _ w401]
              tunnel: w343 -> [_ _ w400]
              frame 17301505 {
                n196 = for {
                  N: 256 -> [_]
                  shift-right: [w391] -> w382
                  shift-left: i32[] [] ("数组") -> [w390]
                  i -> [w387]
                  n197 = Subtract(x=255, y=w387) -> (x-y=w388:i32)
                  n198 = Logical Shift(y=i16 8, x=w388) -> (x << y=w393:i32)
                  n199 = Logical Shift(y=16 ("x"), x=w388) -> (x << y=w394:i32)
                  n200 = Compound Arithmetic op=ADD(w394, w393, w388) -> (w392:i32)
                  n201 = Build Array (concatenate)(w392, w390) -> (w391:i32[])
                }
              }
              frame 35127316 {
              }
              frame Default {
                n202 = Compound Arithmetic op=MULTIPLY(w411, w410, u32 3 ("值")) -> (w408:u32)
                n203 = Bundle By Name(cluster="pConvertInfo In 2", "nWidth"=w403, "nHeight"=w402, "enSrcPixelType"=w401, "nSrcDataLen"=w400, "enDstPixelType"=u32 35127316, "nDstBufferSize"=w408) -> (w407:T5)
                n204 = property on="handle out 2" class="DigNum (strict)"() -> ("Value"=w415:u64)  [unwired: 2 in, 2 out]
                n205 = Initialize Array(u8 0 ("元素"), w408) -> (w413:u8[])
                n206 = call "ConvertPixelType.vi"("handle"=w415, "pSrcData"=w414, "pDstBuf In"=w413, "pConvertInfo In"=w407) -> ("pDstBuf Out"=w404:u8[])  [unwired: 7 in, 4 out]
              }
            }
            n207 = property on="Picture 2" class="Pict"("ZoomFactor"=w359) -> ()  [unwired: 2 in, 2 out]
            n208 = Bundle By Name(cluster="Rectangle 2", "left"=w365, "top"=w365, "right"=w342, "bottom"=w341) -> (w362:T3)
            n209 = Bundle By Name(cluster="image data 2", "image type"=0, "image depth"=w353, "image"=w358, "mask"=u8[] [], "colors"=w357, "Rectangle"=w362) -> (w361:T2)
            n210 = call <vilib>:"Draw Flattened Pixmap.vi"("image data"=w361) -> ("new picture"=→"Picture 2":picture)  [unwired: 8 in]
            "pFrameInfoEx out 2" <- w352
          }
        }
      }
    }
    n211 = case shown="True" w1 {
      frame False {
      }
      frame True {
        n212 = property on="PayloadSize" class="DigNum (strict)"() -> ("Value"=w418:u32)  [unwired: 2 in, 2 out]
        n213 = Wait (ms)(milliseconds to wait=u32 10 ("等待时间（毫秒）")) -> ()  [unwired: 1 out]
        n214 = property on="handle out" class="DigNum (strict)"() -> ("Value"=w421:u64)  [unwired: 2 in, 2 out]
        n215 = Initialize Array(u8 0 ("元素"), w418) -> (w419:u8[])
        n216 = call "GetOneFrameTimeout.vi"("handle"=w421, "pData"=w419, "nDataSize"=w418, "nMsec"=1000) -> ("function return"=w426:i32, "pData Out"=w425:u8[], "pFrameInfoEx out"=w424:T4)  [unwired: 7 in, 2 out]
        n217 = Equal To 0?(x=w426) -> (x = 0?=w428:bool)
        n218 = Initialize Array(u8 0 ("元素"), w418) -> (w422:u8[])
        n219 = case shown="True" w428 {
          tunnel: w425 -> [_ w440]
          tunnel: w424 -> [_ w443]
          tunnel: w422 -> [_ w438]
          frame False {
          }
          frame True {
            w453 = i16 0 ("left")
            n220 = Unbundle By Name(w443) -> ("nWidth"=w435:u16, "nHeight"=w437:u16, "enPixelType"=w430:i32, "nFrameLen"=w439:u32)
            n221 = Compound Arithmetic op=AND(w430, -2147483648 ("value")) -> (w441:i32)
            n222 = case shown="80000000" w441 {
              tunnel: w438 -> [_ w471]
              tunnel: w440 -> [w461 w470]
              tunnel: w439 -> [w458 w469]
              tunnel: [w461 w466] -> w436
              tunnel: [w460 w465] -> w434
              tunnel: [w459 w464] -> w433
              tunnel: [w457 w463] -> w432
              tunnel: [w458 w462] -> w431
              tunnel: w435 -> [w460 _]
              tunnel: w437 -> [w459 _]
              tunnel: w430 -> [w457 _]
              frame Default {
              }
              frame -2147483648 {
                # "HB格式"
                n223 = property on="PayloadSize" class="DigNum (strict)"() -> ("Value"=w468:u32)  [unwired: 2 in, 2 out]
                n224 = property on="handle out" class="DigNum (strict)"() -> ("Value"=w472:u64)  [unwired: 2 in, 2 out]
                n225 = call "HBDecode.vi"("handle"=w472, "pSrcData"=w470, "pDstBuf In"=w471, "SrcDataLen"=w469, "DstBufferSize"=w468) -> ("pDstBuf Out"=w466:u8[], "pHBDecode Out"=w467:T14)  [unwired: 6 in, 3 out]
                n226 = Unbundle By Name(w467) -> ("nWidth"=w465:u32, "nHeight"=w464:u32, "enDstPixelType"=w463:u32, "nDstLen"=w462:u32)
              }
            }
            n227 = property on="Picture" class="Pict"() -> ("Width"=w448:u32)  [unwired: 2 in, 2 out]
            n228 = Divide(x=w448, y=w434) -> (x/y=w447:dbl)
            n229 = case shown="Default" w432 {
              selector: w432 -> [_ _ w493]
              tunnel: w436 -> [w475 w490 w503]
              tunnel: w433 -> [_ _ w491]
              tunnel: w434 -> [_ _ w494]
              tunnel: [w475 w490 w495] -> w446
              tunnel: [8 24 24] -> w444
              tunnel: [w473 i32[] [] i32[] []] -> w445
              tunnel: w431 -> [_ _ w492]
              frame 17301505 {
                n230 = for {
                  N: 256 -> [_]
                  shift-right: [w482] -> w473
                  shift-left: i32[] [] ("数组") -> [w481]
                  i -> [w478]
                  n231 = Subtract(x=255, y=w478) -> (x-y=w479:i32)
                  n232 = Logical Shift(y=i16 8, x=w479) -> (x << y=w484:i32)
                  n233 = Logical Shift(y=16 ("x"), x=w479) -> (x << y=w485:i32)
                  n234 = Compound Arithmetic op=ADD(w485, w484, w479) -> (w483:i32)
                  n235 = Build Array (concatenate)(w483, w481) -> (w482:i32[])
                }
              }
              frame 35127316 {
              }
              frame Default {
                n236 = Compound Arithmetic op=MULTIPLY(w491, w494, u32 3 ("值")) -> (w499:u32)
                n237 = Bundle By Name(cluster="pConvertInfo In", "nWidth"=w494, "nHeight"=w491, "enSrcPixelType"=w493, "nSrcDataLen"=w492, "enDstPixelType"=u32 35127316, "nDstBufferSize"=w499) -> (w498:T5)
                n238 = property on="handle out" class="DigNum (strict)"() -> ("Value"=w504:u64)  [unwired: 2 in, 2 out]
                n239 = Initialize Array(u8 0 ("元素"), w499) -> (w502:u8[])
                n240 = call "ConvertPixelType.vi"("handle"=w504, "pSrcData"=w503, "pDstBuf In"=w502, "pConvertInfo In"=w498) -> ("pDstBuf Out"=w495:u8[])  [unwired: 7 in, 4 out]
              }
            }
            n241 = property on="Picture" class="Pict"("ZoomFactor"=w447) -> ()  [unwired: 2 in, 2 out]
            n242 = Bundle By Name(cluster="Rectangle", "left"=w453, "top"=w453, "right"=w434, "bottom"=w433) -> (w450:T3)
            n243 = Bundle By Name(cluster="image data", "image type"=0, "image depth"=w444, "image"=w446, "mask"=u8[] [], "colors"=w445, "Rectangle"=w450) -> (w449:T2)
            n244 = call <vilib>:"Draw Flattened Pixmap.vi"("image data"=w449) -> ("new picture"=→"Picture":picture)  [unwired: 8 in]
            "pFrameInfoEx out" <- w443
          }
        }
      }
    }
    n245 = event shown="[2] \"stop\": Mouse Down;  Panel Close" {
      selector: _ -> [_ _ _ _ _]
      dyn-events: _ -> [_ _ _ _ _]
      timeout: 10 -> [_ _ _ _ _]
      event Timeout {
        n246 = event-data() -> ()  [unwired: 1 in, 3 out]
      }
      event "Continuous": Mouse Down {
        w5 = T8."Disabled and Grayed Out" ("禁用")
        n247 = event-data() -> ()  [unwired: 1 in, 8 out]
        n248 = property on="handle out 2" class="DigNum (strict)"() -> ("Value"=w13:u64)  [unwired: 2 in, 2 out]
        n249 = property on="handle out" class="DigNum (strict)"() -> ("Value"=w6:u64)  [unwired: 2 in, 2 out]
        n250 = call "SetEnumValue.vi"("nValue"=u32 0, "strKey"="TriggerMode", "handle"=w13) -> ()  [unwired: 6 in, 3 out]
        n251 = call "SetEnumValue.vi"("nValue"=u32 0, "strKey"="TriggerMode", "handle"=w6) -> ("error out"=w7:errorcluster)  [unwired: 6 in, 2 out]
        n252 = property on="Continuous" class="Bool"(error in=w7, "DisabledEnum"=w5) -> (error out=w10:errorcluster)  [unwired: 1 in, 1 out]
        n253 = property on="Trigger Mode" class="Bool"(error in=w10, "DisabledEnum"=T8."Enabled" ("禁用")) -> (error out=w8:errorcluster)  [unwired: 1 in, 1 out]
        n254 = property on="Trigger Once" class="Bool"(error in=w8, "DisabledEnum"=w5) -> ()  [unwired: 1 in, 2 out]
      }
      event "stop": Mouse Down; Panel Close {
        n255 = event-data() -> ()  [unwired: 1 in, 3 out]
        n256 = flat-sequence {
          frame #0 {
            n257 = property on="打开标志" class="Bool (strict)"("Value"=FALSE ("打开标志")) -> (error out=w18:errorcluster)  [unwired: 2 in, 1 out]
            n258 = property on="Acquisision Flag" class="Bool (strict)"(error in=w18, "Value"=FALSE ("采集标志")) -> (error out=w16:errorcluster)  [unwired: 1 in, 1 out]
            n259 = property on="handle out 2" class="DigNum (strict)"(error in=w16) -> ("Value"=w22:u64)  [unwired: 1 in, 2 out]
            n260 = property on="handle out" class="DigNum (strict)"(error in=w16) -> ("Value"=w17:u64)  [unwired: 1 in, 2 out]
            n261 = property on="打开标志" class="Bool (strict)"() -> ("Value"=w23:bool)  [unwired: 2 in, 2 out]
            n262 = property on="打开标志" class="Bool (strict)"() -> ("Value"=w21:bool)  [unwired: 2 in, 2 out]
            n263 = case shown="True" w23 {
              tunnel: w22 -> [_ w28]
              frame False {
              }
              frame True {
                n264 = call "CloseDevice.vi"("handle"=w28) -> ("error out"=w29:errorcluster, "handle out"=w27:u64)  [unwired: 8 in, 1 out]
                n265 = call "DestroyHandle.vi"("error in (no error)"=w29, "handle"=w27) -> ()  [unwired: 8 in, 2 out]
              }
            }
            n266 = case shown="True" w21 {
              tunnel: w17 -> [_ w25]
              frame False {
              }
              frame True {
                n267 = call "CloseDevice.vi"("handle"=w25) -> ("error out"=w26:errorcluster, "handle out"=w24:u64)  [unwired: 8 in, 1 out]
                n268 = call "DestroyHandle.vi"("error in (no error)"=w26, "handle"=w24) -> ()  [unwired: 8 in, 2 out]
              }
            }
          }
          frame #1 {
            n269 = call "Finalize.vi"() -> ()  [unwired: 10 in, 2 out]
          }
          frame #2 {
            n270 = property on="Open Device" class="Bool"("DisabledEnum"=T8."Enabled" ("禁用")) -> ()  [unwired: 2 in, 2 out]
            n271 = property on="Close Device" class="Bool"("DisabledEnum"=T8."Disabled and Grayed Out" ("禁用")) -> ()  [unwired: 2 in, 2 out]
            n272 = property on="Trigger Once" class="Bool"("DisabledEnum"=T8."Disabled and Grayed Out" ("禁用")) -> ()  [unwired: 2 in, 2 out]
            n273 = property on="Start" class="Bool"("DisabledEnum"=T8."Disabled and Grayed Out" ("禁用")) -> ()  [unwired: 2 in, 2 out]
            n274 = property on="Stop" class="Bool"("DisabledEnum"=T8."Disabled and Grayed Out" ("禁用")) -> ()  [unwired: 2 in, 2 out]
            n275 = property on="Continuous" class="Bool"("DisabledEnum"=T8."Disabled and Grayed Out" ("禁用")) -> ()  [unwired: 2 in, 2 out]
            n276 = property on="Trigger Mode" class="Bool"("DisabledEnum"=T8."Disabled and Grayed Out" ("禁用")) -> ()  [unwired: 2 in, 2 out]
          }
        }
      }
      event "Trigger Mode": Mouse Down {
        n277 = event-data() -> ()  [unwired: 1 in, 8 out]
        n278 = property on="handle out 2" class="DigNum (strict)"() -> ("Value"=w44:u64)  [unwired: 2 in, 2 out]
        n279 = property on="handle out" class="DigNum (strict)"() -> ("Value"=w38:u64)  [unwired: 2 in, 2 out]
        n280 = call "SetEnumValue.vi"("nValue"=u32 1, "strKey"="TriggerMode", "handle"=w44) -> ("error out"=w48:errorcluster)  [unwired: 6 in, 2 out]
        n281 = call "SetEnumValue.vi"("nValue"=u32 1, "strKey"="TriggerMode", "handle"=w38) -> ("error out"=w39:errorcluster)  [unwired: 6 in, 2 out]
        n282 = call "SetEnumValue.vi"("error in (no error)"=w39, "nValue"=u32 7, "strKey"="TriggerSource", "handle"=w38) -> ()  [unwired: 5 in, 3 out]
        n283 = call "SetEnumValue.vi"("error in (no error)"=w48, "nValue"=u32 7, "strKey"="TriggerSource", "handle"=w44) -> ("error out"=w37:errorcluster)  [unwired: 5 in, 2 out]
        n284 = property on="Trigger Mode" class="Bool"(error in=w37, "DisabledEnum"=T8."Disabled and Grayed Out" ("禁用")) -> ()  [unwired: 1 in, 2 out]
        n285 = property on="Continuous" class="Bool"(error in=w37, "DisabledEnum"=T8."Enabled" ("禁用")) -> ()  [unwired: 1 in, 2 out]
        n286 = property on="Trigger Once" class="Bool"(error in=w37, "DisabledEnum"=T8."Enabled" ("禁用")) -> ()  [unwired: 1 in, 2 out]
      }
      event "Trigger Once": Mouse Down {
        n287 = event-data() -> ()  [unwired: 1 in, 8 out]
        n288 = property on="handle out 2" class="DigNum (strict)"() -> ("Value"=w53:u64)  [unwired: 2 in, 2 out]
        n289 = property on="handle out" class="DigNum (strict)"() -> ("Value"=w57:u64)  [unwired: 2 in, 2 out]
        n290 = call "SetCommandValue.vi"("strValue"="TriggerSoftware", "handle"=w57) -> ("function return"=w59:i32)  [unwired: 7 in, 2 out]
        n291 = call "SetCommandValue.vi"("strValue"="TriggerSoftware", "handle"=w53) -> ("function return"=w55:i32)  [unwired: 7 in, 2 out]
        n292 = Equal To 0?(x=w59) -> (x = 0?=w58:bool)
        n293 = Equal To 0?(x=w55) -> (x = 0?=w54:bool)
        n294 = case shown="False" w58 {
          frame False {
            n295 = One Button Dialog(message="Trigger Cam1 Failed") -> ()  [unwired: 1 in, 1 out]
          }
          frame True {
            n296 = One Button Dialog(message="Trigger Can1 Success") -> ()  [unwired: 1 in, 1 out]
          }
        }
        n297 = case shown="False" w54 {
          frame False {
            n298 = One Button Dialog(message="Trigger Cam2 Failed") -> ()  [unwired: 1 in, 1 out]
          }
          frame True {
            n299 = One Button Dialog(message="Trigger Cam2 Success") -> ()  [unwired: 1 in, 1 out]
          }
        }
      }
    }
  }
